vi "扭矩.vi"   [LabVIEW 2020]
uses:
  <userlib>/DAQNavi Polymorphic VI/create/DAQNavi Create Channel(AI-Voltage).vi
  Global_Variable/Global.vi
  <userlib>/DAQNavi Polymorphic VI/read/DAQNavi Read (Analog 1D DBL NChan 1Samp).vi
  Global_Variable/excursion.vi
  <userlib>/_MGI/1D Array/MGI Running Average/MGI Running Average(DBL).vi
  <vilib>/ptbypt/NI_PtbyPt.lvlib
types:
  T1 = cluster{"右正向":dbl, "右逆向":dbl, "左正向":dbl, "左逆向":dbl}
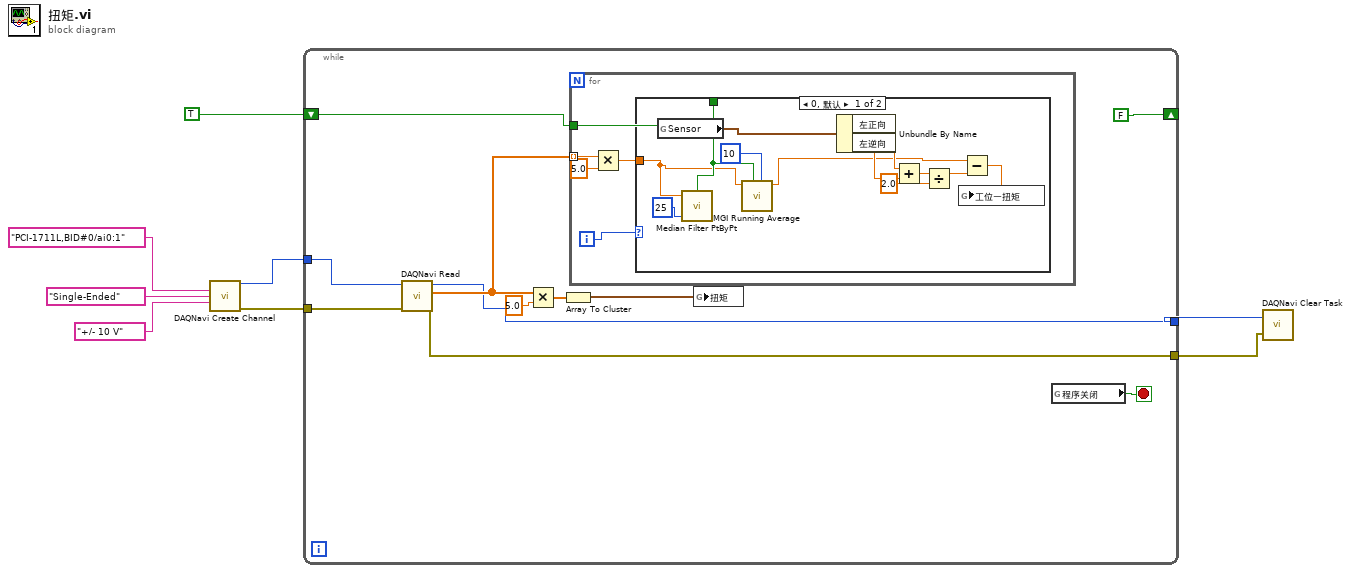
[diagram p0: block diagram]
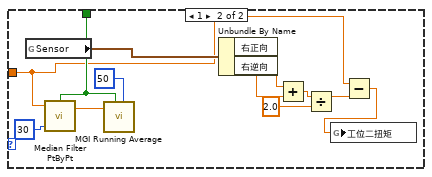
[diagram p2: hidden frame]
diagram:
  n1 = call-poly <userlib>:"DAQNavi Create Channel.vi"("physical channels"="PCI-1711L,BID#0/ai0:1", "signal type"="Single-Ended", "value range"="+/- 10 V") -> ("task out"=w6:i32, "error out"=w5:errorcluster)  [unwired: 11 in]
  n2 = while {
    tunnel: w6 -> [w19]
    tunnel: w5 -> [w18]
    shift-right: [FALSE] -> _
    shift-left: TRUE -> [w11]
    tunnel: [w10] -> w2
    tunnel: [w9] -> w1
    stop <- w16 stop-if-true
    n3 = call-poly <userlib>:"DAQNavi Read.vi"("error in (no error)"=w18, "task in"=w19) -> ("error out"=w9:errorcluster, "data"=w13:dbl[], "task out"=w10:i32)  [unwired: 7 in]
    n4 = Multiply(x=w13, y=5.0) -> (x*y=w15:dbl[])
    n5 = Array To Cluster(array=w15) -> (cluster=w14:cluster{"[0]":dbl, "[1]":dbl})
    n6 = for {
      tunnel: w13 -> [w22] mode=indexing
      tunnel: w11 -> [w20]
      i -> [w24]
      n7 = Multiply(x=w22, y=5.0) -> (x*y=w21:dbl)
      n8 = case shown="0, 默认" w24 {
        tunnel: w21 -> [w26 w37]
        tunnel: w20 -> [w35 w48]
        frame 0, Default {
          n9 = global read "excursion.vi" "Sensor"() -> (w25:T1)
          n10 = call <vilib>:"Median Filter PtByPt.vi"("initialize"=w35, "rank"=25, "x"=w26) -> ()  [unwired: 1 in, 2 out]
          n11 = call-poly <userlib>:"MGI Running Average.vi"("Averaging Size"=10, "Initialize? (F)"=w35, "Value"=w26) -> ("Average"=w28:dbl)  [unwired: 8 in]
          n12 = Unbundle By Name(w25) -> ("左正向"=w33:dbl, "左逆向"=w32:dbl)
          n13 = Add(x=w33, y=w32) -> (x+y=w31:dbl)
          n14 = Divide(x=w31, y=2.0) -> (x/y=w30:dbl)
          n15 = Subtract(x=w28, y=w30) -> (x-y=w27:dbl)
          n16 = global write "Global.vi" "工位一扭矩"(w27) -> ()
        }
        frame 1 {
          n17 = global read "excursion.vi" "Sensor"() -> (w39:T1)
          n18 = call <vilib>:"Median Filter PtByPt.vi"("initialize"=w48, "rank"=30, "x"=w37) -> ("Filtered x"=w38:dbl)  [unwired: 1 in, 1 out]
          n19 = call-poly <userlib>:"MGI Running Average.vi"("Averaging Size"=50, "Initialize? (F)"=w48, "Value"=w38) -> ()  [unwired: 8 in, 1 out]
          n20 = Unbundle By Name(w39) -> ("右正向"=w45:dbl, "右逆向"=w44:dbl)
          n21 = Add(x=w45, y=w44) -> (x+y=w43:dbl)
          n22 = Divide(x=w43, y=2.0) -> (x/y=w42:dbl)
          n23 = Subtract(x=w37, y=w42) -> (x-y=w40:dbl)
          n24 = global write "Global.vi" "工位二扭矩"(w40) -> ()
        }
      }
    }
    n25 = global write "Global.vi" "扭矩"(w14) -> ()
    n26 = global read "Global.vi" "程序关闭"() -> (w16:bool)
  }
  n27 = call <userlib>:"DAQNavi Clear Task.vi"("error in (no error)"=w1, "task in"=w2) -> ()  [unwired: 1 in, 1 out]
